vi "StringTo1DSGL.vi"(0 "String":string, 7 "Offset":i32 caption="Offset (0)", 11 "Error in":errorcluster caption="Error in (no error)") -> (4 "Array":sgl[](array[numeric]), 8 "Offset Past Array":i32, 15 "Error out":errorcluster)   [LabVIEW 2017, in "GPString.lvlib"]
doc: "Converts <B>String</B> to <B>Array</B>, starting the conversion from the optional <B>Offset</B> in <B>String</B>.\n\n<B>String formatting</B>\n- Both period (.) and comma (,) are supported as radix point in the numbers in <B>String</B>.\n- Element separator character must be \";\".\n- Array enclosure characters can be either square or curly brackets.\n\nThis VI is inlined.\n\nSteen Schmidt\nGPower\n15/6 2016"
uses:
  GPString.lvlib
panel:
  # "Copyright © 2016\nGPower\nSee enclosed license file for terms and conditions"
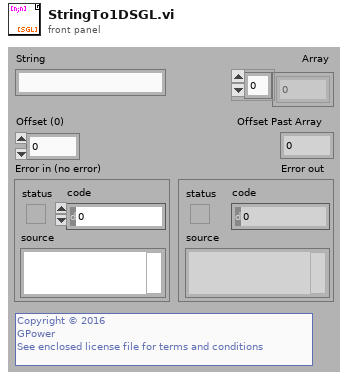
[diagram p1: front panel]
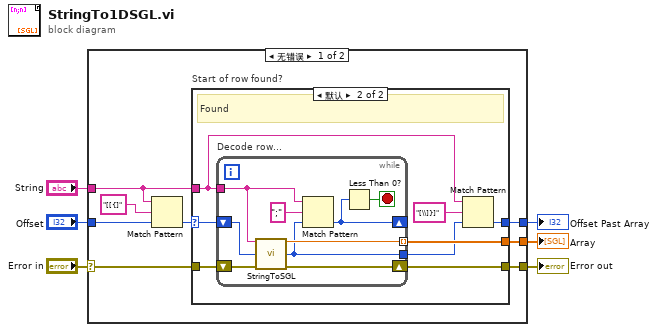
[diagram p0: block diagram]
diagram:
  n1 = case shown="无错误" "Error in" {
    selector: "Error in" -> [w11 w35]
    tunnel: "String" -> [w9 _]
    tunnel: "Offset" -> [w7 w34]
    tunnel: [w13 _] -> w4
    tunnel: [w12 w35] -> w3
    tunnel: [w10 w34] -> w1
    frame No Error {
      n2 = Match Pattern(string=w9, regular expression="[[{]", offset (0)=w7) -> (offset past match=w8:i32)  [unwired: 3 out]
      n3 = case "Start of row found?" shown="默认" w8 {
        selector: w8 -> [w15 w17]
        tunnel: [_ w24] -> w13
        tunnel: [w16 w23] -> w12
        tunnel: w11 -> [w16 w22]
        tunnel: [w15 w20] -> w10
        tunnel: w9 -> [_ w18]
        frame -1 {
          # "Not found"
        }
        frame Default {
          # "Found"
          n4 = while "Decode row..." {
            tunnel: w18 -> [w30]
            shift-right: [w27] -> _
            shift-left: w17 -> [w29]
            shift-right: [w28] -> w23
            shift-left: w22 -> [w33]
            tunnel: [w32] -> w24 mode=indexing
            tunnel: [w25] -> w19
            stop <- w26 stop-if-true
            n5 = call "StringToSGL.vi"("String"=w30, "Offset"=w29, "Error in"=w33) -> ("Number"=w32:sgl, "Offset Past Number"=w25:i32, "Error out"=w28:errorcluster)  [unwired: 10 in]
            n6 = Match Pattern(string=w30, regular expression=";", offset (0)=w25) -> (offset past match=w27:i32)  [unwired: 3 out]
            n7 = Less Than 0?(x=w27) -> (x < 0?=w26:bool)
          }
          n8 = Match Pattern(string=w18, regular expression="[\\]}]", offset (0)=w19) -> (offset past match=w20:i32)  [unwired: 3 out]
        }
      }
    }
    frame Error {
    }
  }
  "Array" <- w4
  "Error out" <- w3
  "Offset Past Array" <- w1
